vi "WAV_read.vi"(11 "file (use dialog)":path) -> (0 "error out":errorcluster, 1 "Valid?":bool, 2 "File Size":u32, 3 "string out":string)   [LabVIEW 2022 SP3]
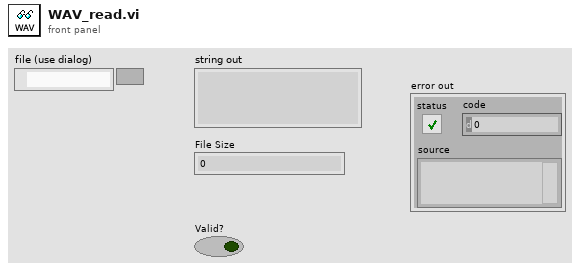
[diagram p1: front panel]
types:
  T1 = enum16{"big-endian, network order", "native, host order", "little-endian"}
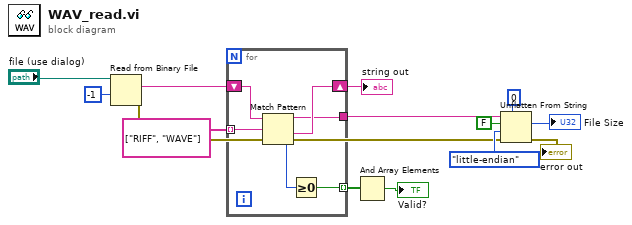
[diagram p0: block diagram]
diagram:
  n1 = Read from Binary File(10:-1 ("count (1)"), 11:"file (use dialog)") -> (0:w2:errorcluster, 2:w5:string)  [unwired: 4 in, 2 out]
  n2 = for {
    tunnel: string[] ["RIFF", "WAVE"] -> [w20] mode=indexing
    shift-right: [w19] -> w7
    shift-left: w5 -> [w18]
    tunnel: [w17] -> w11
    tunnel: [w15] -> w6 mode=indexing
    n3 = Match Pattern(string=w18, regular expression=w20) -> (before substring=w17:string, after substring=w19:string, offset past match=w16:i32)  [unwired: 1 in, 1 out]
    n4 = Greater Or Equal To 0?(x=w16) -> (x >= 0?=w15:bool)
  }
  "string out" <- w7
  n5 = And Array Elements(Boolean array=w6) -> (logical AND=→"Valid?":bool)
  n6 = Unflatten From String(type=u32 0 ("count"), binary string=w11, data includes array or string size? (T)=FALSE, byte order (0:big-endian, network order)=T1."little-endian", error in (no error)=w2) -> (value=→"File Size":u32, error out=→"error out":errorcluster)  [unwired: 1 out]
